vi "multifit_old.vi"(6 "error in":errorcluster, 8 "List Peaks":string[][](table)=[["0", "2.298448", "56622.259938"], ["1", "3.693510", "568942.221745"], ["2", "3.986486", "85674.157303"], ["3", "12.564011", "20786.516854"]], 9 "List Parameter Fit In":dbl[][](array[numeric])=[[61895.26743495138, 2.295902819051137, 0.05132725028401794, 4549.770440475167, 604.272909684641, 0.00013211395312335064, 0.0005412786405150726, 657.5539740905274], [627372.2059878254, 3.692284511840813, 0.05677911685996556, 18601.27709030301, 3836.7824698281233, 8.354403497208279e-05, 0.0003643877607762332, 4160.712473210559], [74116.31578446296, 4.0147483591783155, 0.05085091795005294, 22427.950314927708, 307.3617647197942, 0.00014015981359792937, 0.0002809232075470725, 309.9731656877187], [28273.34836642687, 12.573977083982806, 0.10770256815937904, 51.48314892156685, 1352.5083475039019, 0.0004671472170224425, 0.004032939443201791, 1403.8484860391175]], 10 "List ROI In":dbl[][](array[numeric])=[[2.295902819051137, 0.12087567441886224, 747.0, 785.0, 2.233926550867361, 2.356038682169207, 6063.6329279938445, 123.14309366808929], [3.692284511840813, 0.1337148202052189, 1180.0, 1222.0, 3.625362152280503, 3.760328192140438, 67989.42495261344, 852.13028597231], [4.0147483591783155, 0.11975391177237468, 1283.0, 1320.0, 3.956350297651297, 4.075248951813621, 7193.497223633383, 69.57166423918198], [12.573977083982806, 0.2536395480153376, 3925.0, 4004.0, 12.446356900269128, 12.700221594291389, 5812.069028071378, 495.66499136986374]], 11 "Spectrum In":cluster{"Locations":dbl[], "Amplitudes":dbl[]}={"Locations"=array[8192 elements], "Amplitudes"=array[8192 elements]}) -> (1 "List Parameter Fit Out":dbl[][](array[numeric])=[[72985.42049784464, 2.29530433588858, 0.05722471236395812, -6719.954128683837, 3514.3279732857486, 7.641139969591555e-05, 0.0017646666004499732, 3559.3620345490303], [626906.4516896611, 3.6923878537448513, 0.056725550141628785, 19143.182126509742, 2756.558061175683, 9.742740047455971e-05, 0.00030585131086768315, 3020.7605065816324], [84952.09034117158, 4.0147539339226315, 0.05684400456146576, 11048.984691445543, 3382.5195465814695, 5.6421783276986587e-05, 0.0014333924536871097, 3422.1830799296517]], 2 "List ROI Out":dbl[][](array[numeric])=[[2.29530433588858, 0.13476419761712136, 745.0, 787.0, 2.2274995965883164, 2.3624656364482517, 7971.631104776367, 629.6678820155158], [3.6923878537448513, 0.1335886705835358, 1180.0, 1222.0, 3.625362152280503, 3.760328192140438, 67874.85518278569, 664.4170311995598], [4.0147539339226315, 0.13386763074225186, 1280.0, 1322.0, 3.9467098662327302, 4.0816759060926655, 9216.928010954993, 599.404820008226]], 3 "Spectrum Fitted":cluster{"Array":dbl[], "Array":dbl[]}, 4 "error out":errorcluster)   [LabVIEW 2020]
uses:
  <vilib>/Analysis/6fits.llb/Curve Fitting Criteria.ctl
  <vilib>/gmath/NumericalOptimization/Nonlinear Curve Fit LM bound.vi
  <vilib>/gmath/NI_Gmath.lvlib
  <vilib>/gmath/NumericalOptimization/Nonlinear Curve Fit LM.vi
  <vilib>/Analysis/NI_AALPro.lvlib
panel:
  in  "FWHM Bound Parameters (%)":dbl=60.0
  out "List MultiFit":dbl[][](array[numeric])
  out "R-square":dbl
  out "All FWHM":dbl[](array[numeric])
  out "All Parameters Fit":T1(array[cluster])
  in  "EnOffsetFit":bool
  in  "Erase":bool
  in  "List Fit Peak":T2(array[cluster])
  in  "mapping":u16(ring) items=["Y - Linear", "Y - Log"]
  in  "Fit":bool
  in  "Done":bool
  out "Spectrum":T3(graph)
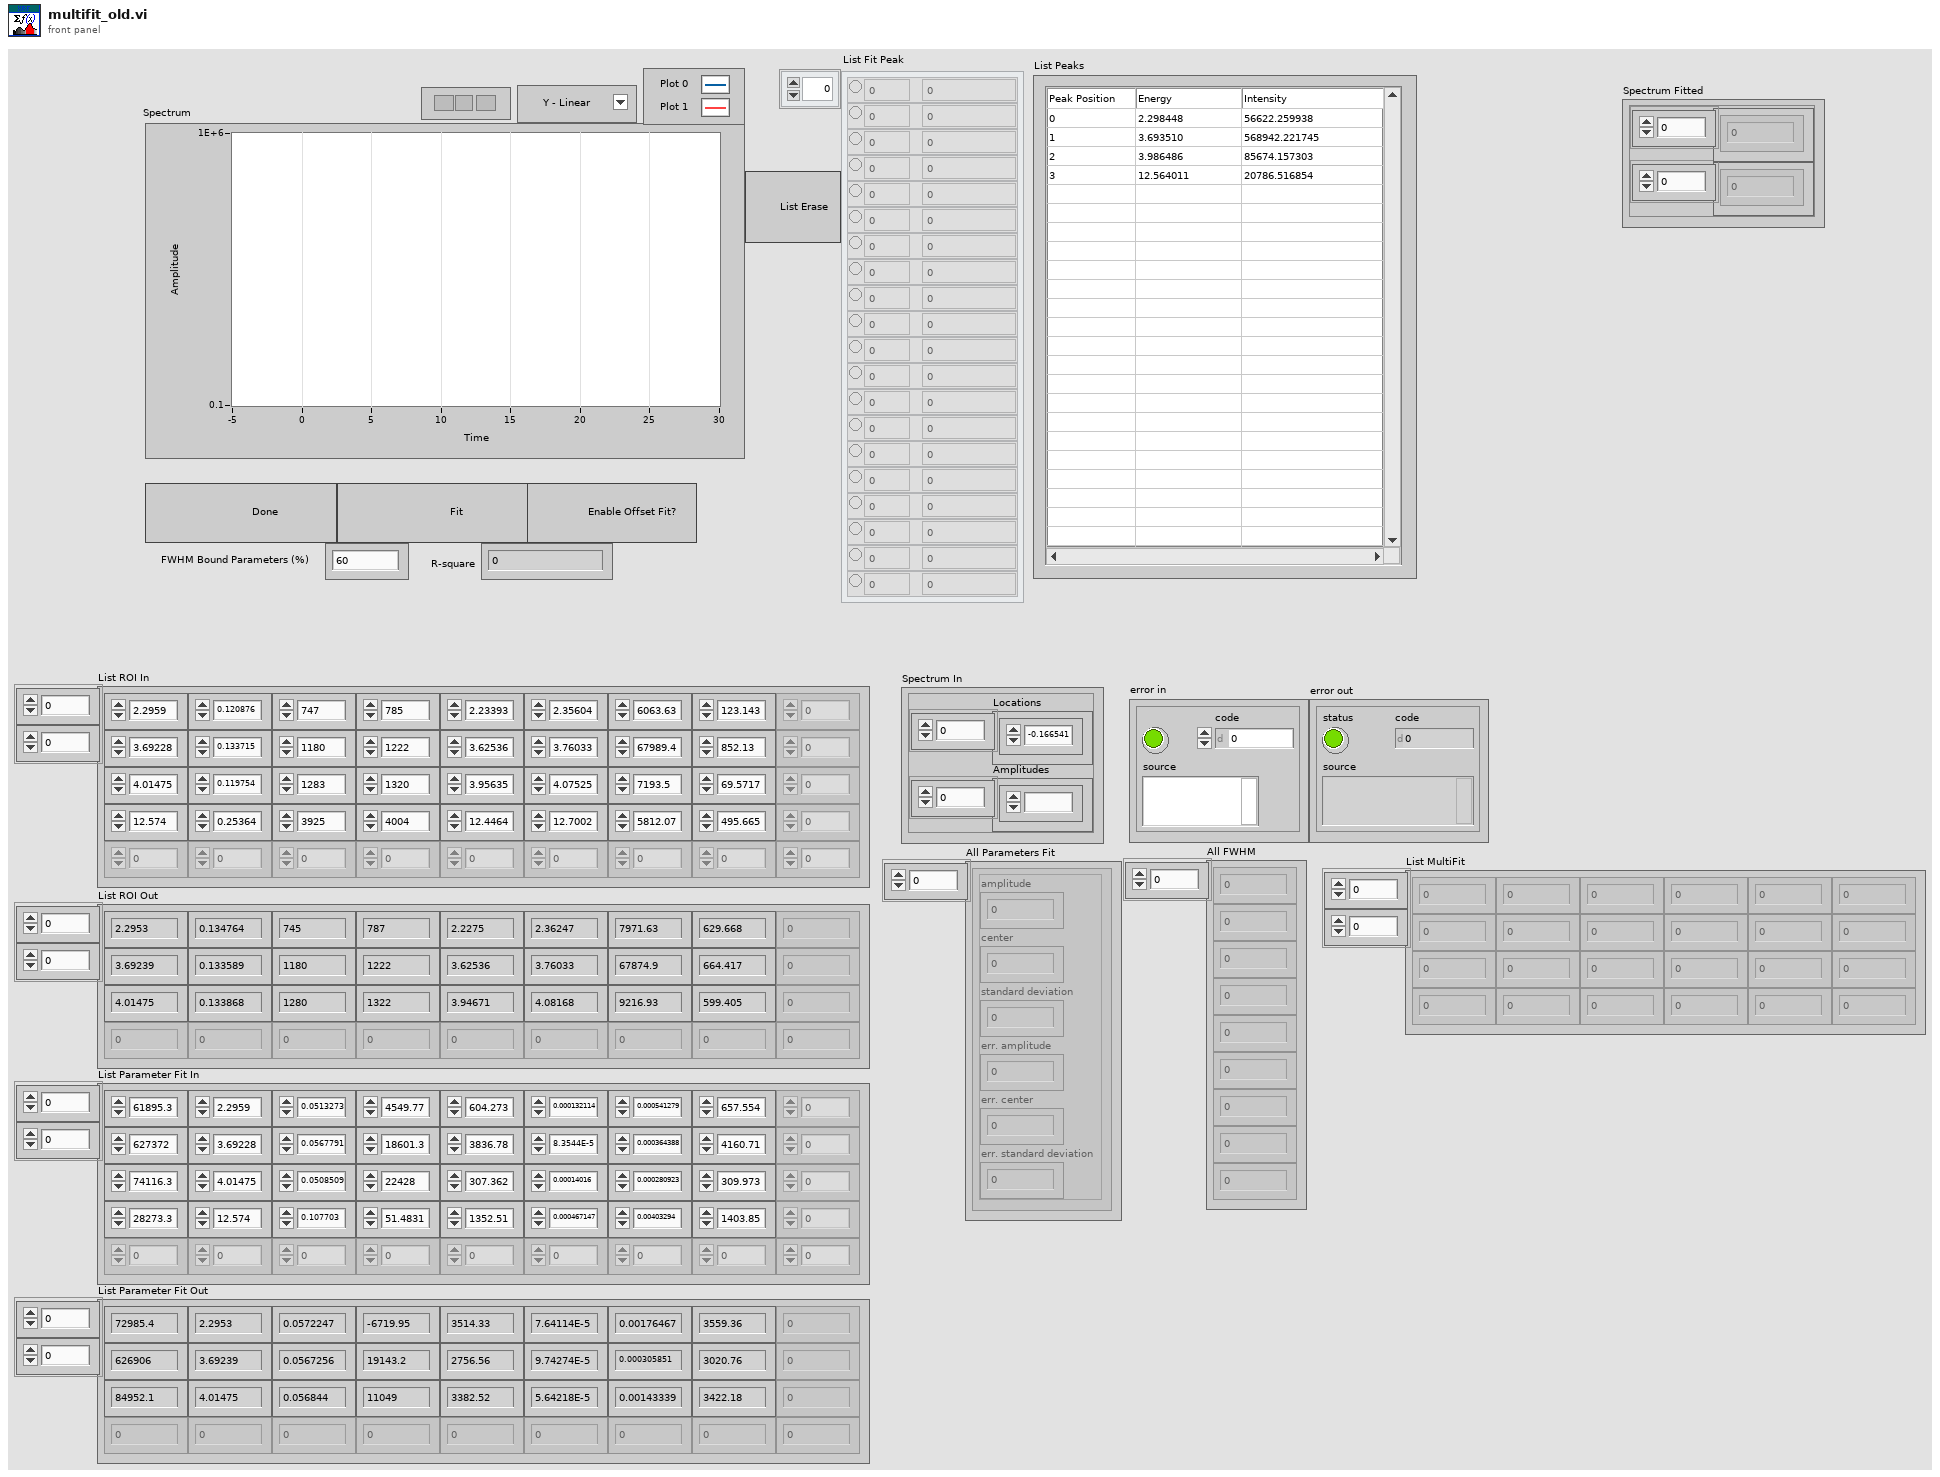
[diagram p1: front panel]
types:
  T1 = cluster{"amplitude":dbl, "center":dbl, "standard deviation":dbl, "err. amplitude":dbl, "err. center":dbl, "err. standard deviation":dbl}[]
  T2 = cluster{"Include":bool, "Position":dbl, "Energy":dbl}[]
  T3 = cluster{"Locations":dbl[], "best nonlinear fit":dbl[]}[]
  T4 = cluster{"Include":bool, "Position":dbl, "Energy":dbl}
  T5 = cluster{"parameter minimum":dbl[], "parameter maximum":dbl[]}
  T6 = typedef "NI_AALPro.lvlib/Curve Fitting Criteria.ctl" = u16
  T7 = typedef "NI_Matrix.lvlib/RealMatrix.ctl" = dbl[][]
  T8 = cluster{"Locations":dbl[], "best nonlinear fit":dbl[]}
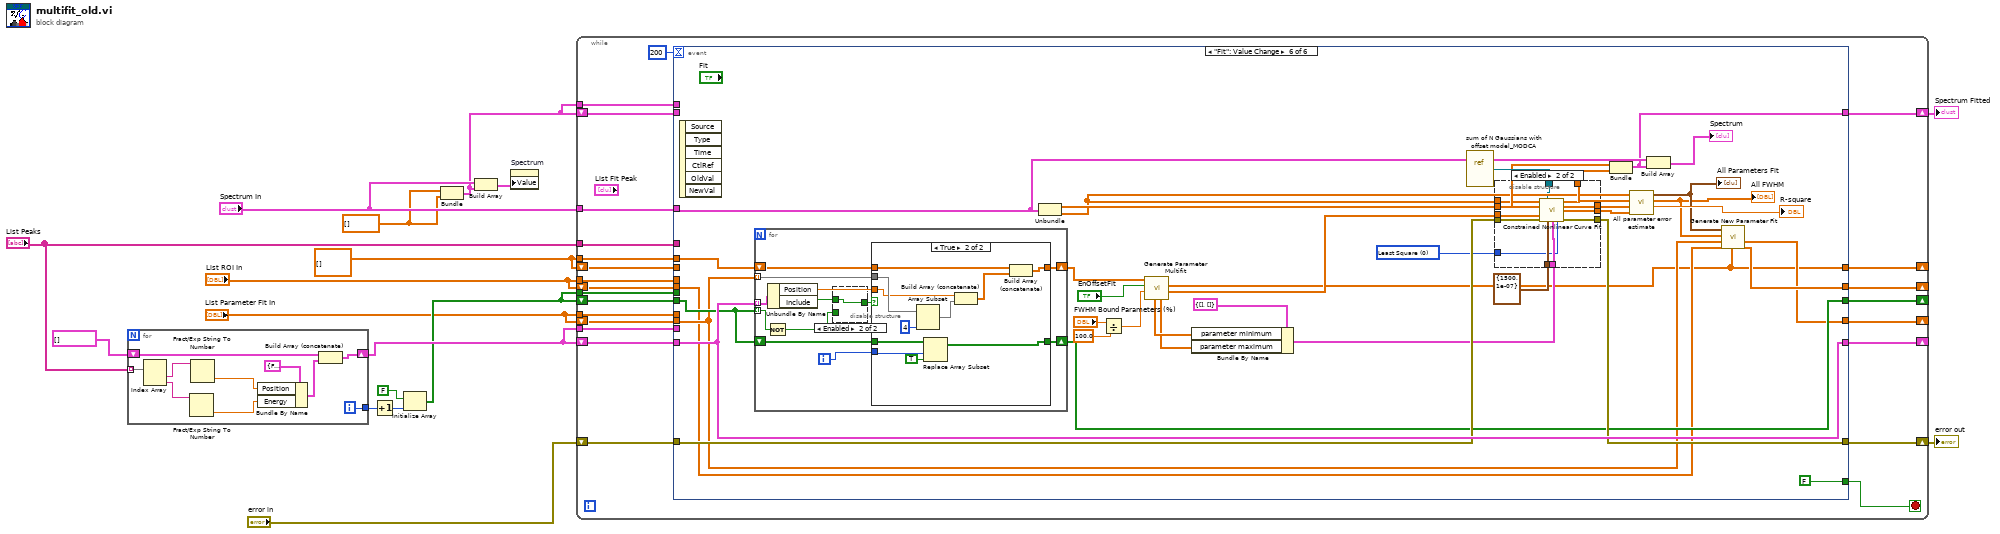
[diagram p0: block diagram]
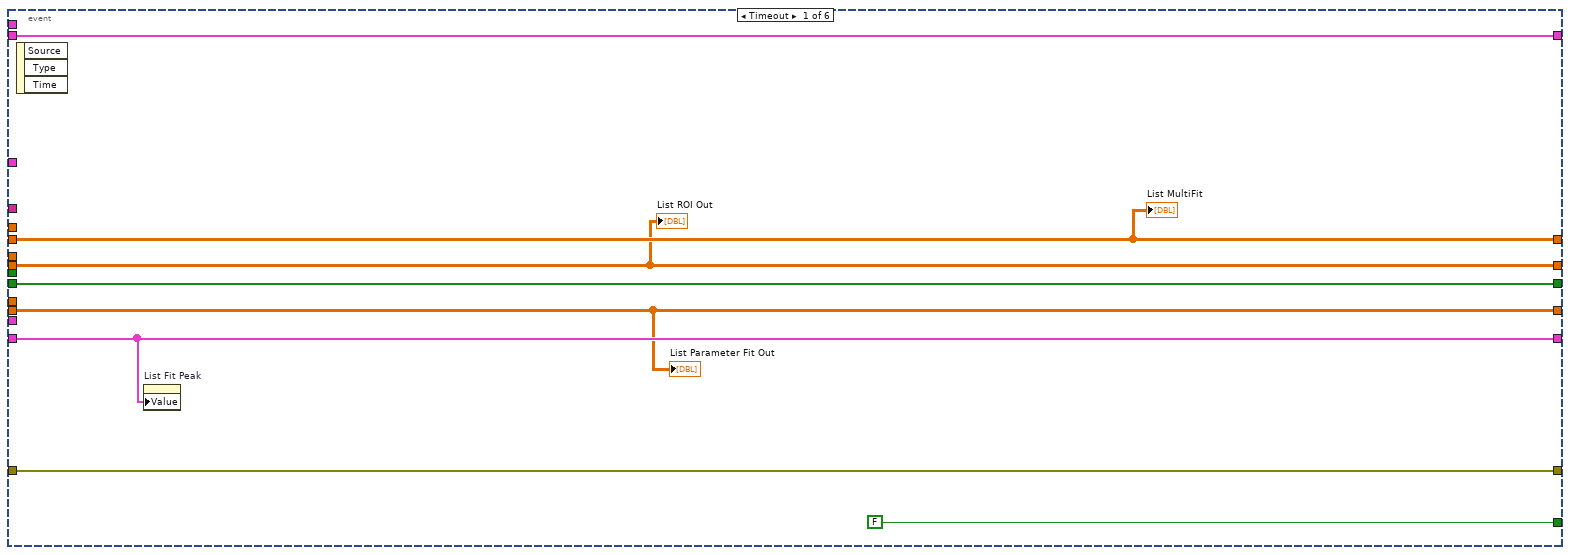
[diagram p2: hidden frame]
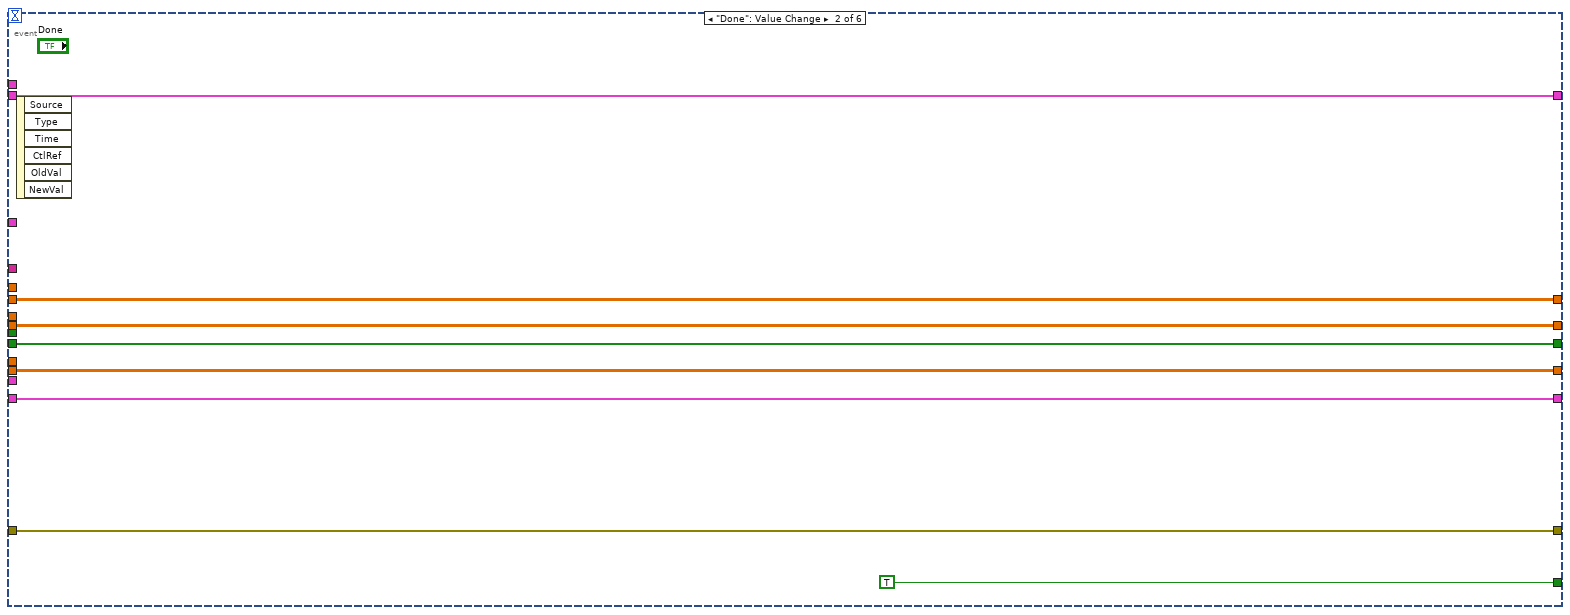
[diagram p3: hidden frame]
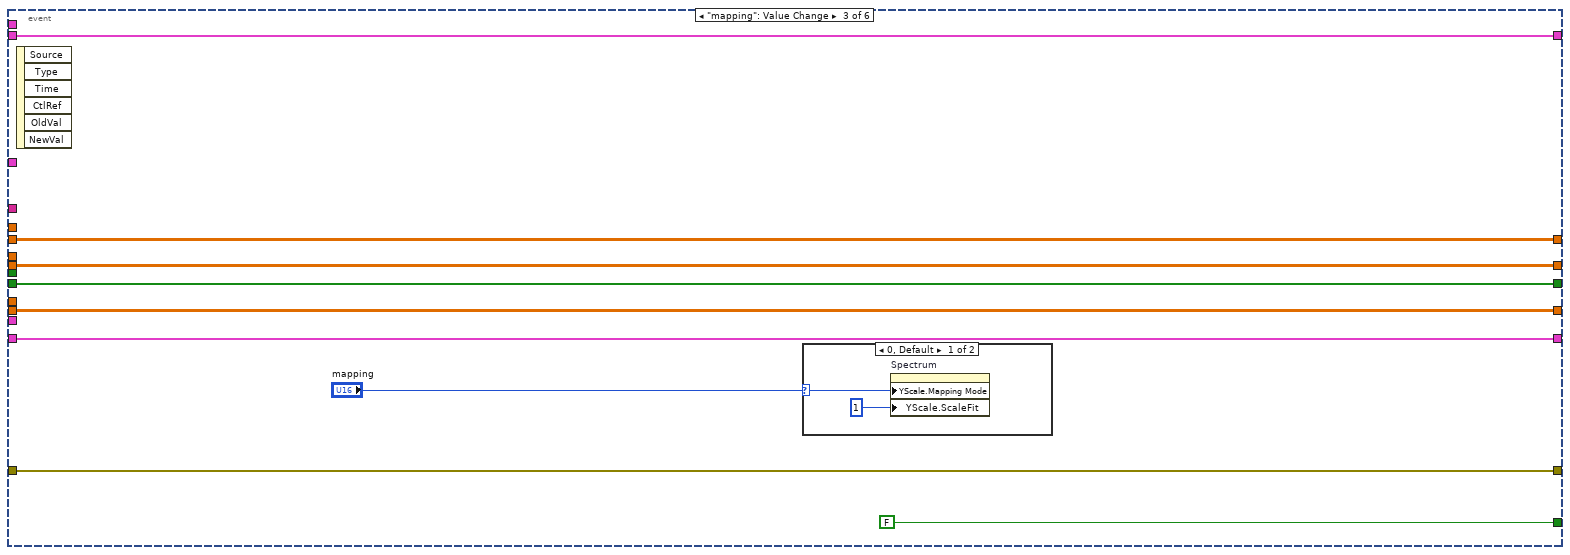
[diagram p4: hidden frame]
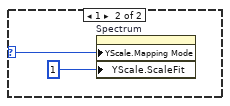
[diagram p5: hidden frame]
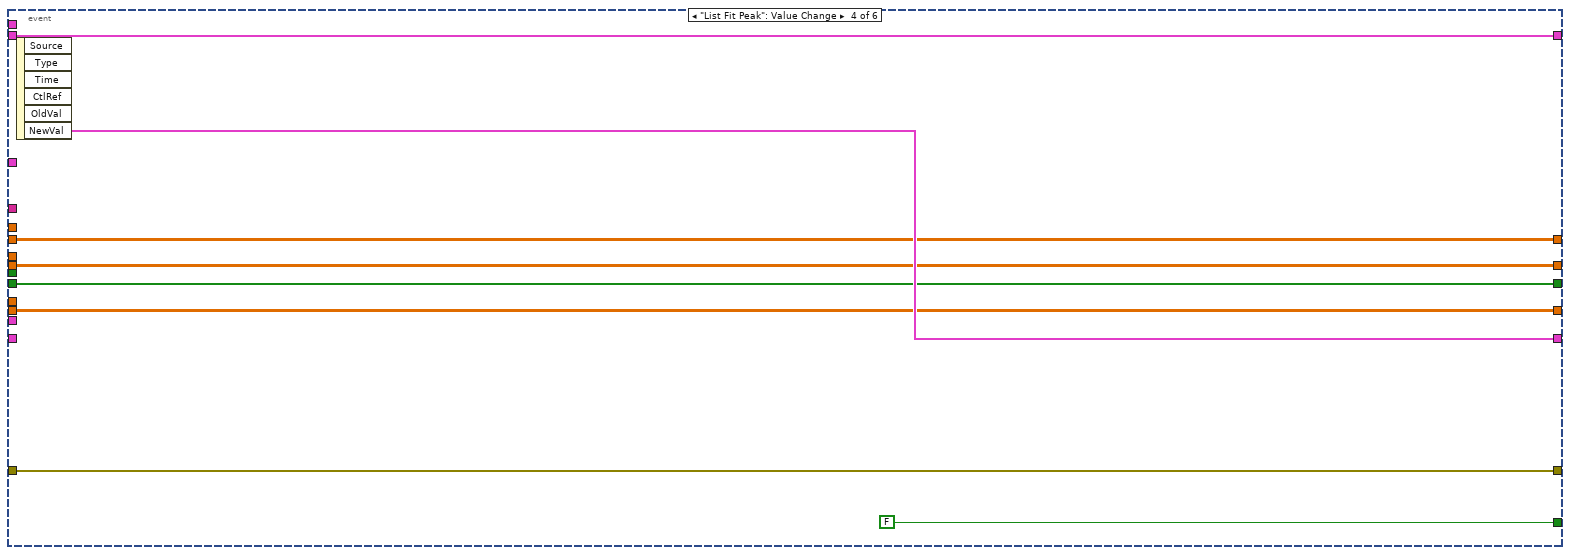
[diagram p6: hidden frame]
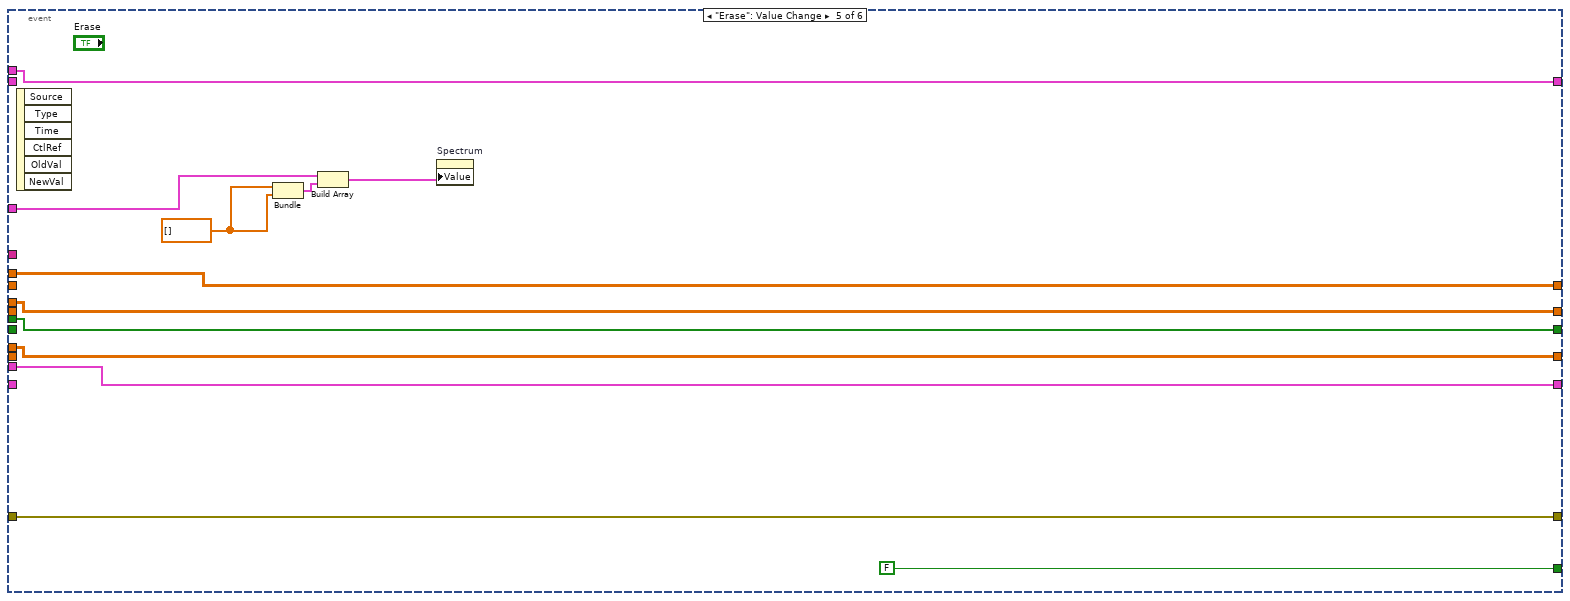
[diagram p7: hidden frame]
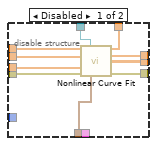
[diagram p8: hidden frame]
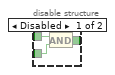
[diagram p9: hidden frame]
diagram:
  w5 = dbl[] []
  w8 = dbl[][] [] ("List ROI In")
  n1 = for {
    tunnel: "List Peaks" -> [w27] mode=indexing
    shift-right: [w23] -> w13
    shift-left: T2 [] ("List Peak") -> [w25]
    tunnel: [w18] -> w12
    i -> [w18]
    n2 = Index Array(array=w27) -> (element #1=w22:string, element #2=w21:string)  [unwired: 2 in]
    n3 = Fract/Exp String To Number(string=w21) -> (number=w19:dbl)  [unwired: 3 in, 1 out]
    n4 = Fract/Exp String To Number(string=w22) -> (number=w20:dbl)  [unwired: 3 in, 1 out]
    n5 = Bundle By Name(cluster=T4 {"Include"=FALSE, "Position"=0.0, "Energy"=0.0} ("Fit Peak Cluster"), "Position"=w20, "Energy"=w19) -> (w24:T4)
    n6 = Build Array (concatenate)(w25, w24) -> (w23:T2)
  }
  n7 = Increment(x=w12) -> (x+1=w11:i32)
  n8 = Initialize Array(FALSE, w11) -> (w9:bool[])
  n9 = Bundle(w5, w5) -> (w2:cluster{dbl[], dbl[]})  [unwired: 1 in]
  n10 = Build Array("Spectrum In", w2) -> (w7:cluster{"Locations":dbl[], "Amplitudes":dbl[]}[])
  n11 = property on="Spectrum" class="XYGraph (strict)"("Value"=w7) -> ()  [unwired: 2 in, 2 out]
  n12 = while {
    shift-right: [w49] -> w16
    shift-left: "error in" -> [w50]
    shift-right: [w47] -> _
    shift-left: w13 -> [w48]
    tunnel: "Spectrum In" -> [w45]
    tunnel: "List Peaks" -> [w44]
    tunnel: "List ROI In" -> [w43]
    tunnel: "List Parameter Fit In" -> [w42]
    tunnel: w13 -> [w41]
    shift-right: [w39] -> _
    shift-left: w8 -> [w40]
    shift-right: [w38] -> _
    shift-left: w9 -> [w37]
    tunnel: w9 -> [w36]
    tunnel: w8 -> [w35]
    shift-right: [w32] -> _
    shift-left: "List ROI In" -> [w34]
    shift-right: [w31] -> _
    shift-left: "List Parameter Fit In" -> [w33]
    shift-right: [w30] -> w1
    shift-left: w2 -> [w29]
    tunnel: w2 -> [w28]
    stop <- w51 stop-if-true
    n13 = event shown="[5] \"Fit\": Value Change" {
      selector: _ -> [_ _ _ _ _ _]
      dyn-events: _ -> [_ _ _ _ _ _]
      timeout: 200 -> [_ _ _ _ _ _]
      tunnel: [FALSE TRUE FALSE FALSE FALSE FALSE] -> w51
      tunnel: w50 -> [w58 w66 w74 w88 w99 w134]
      tunnel: [w58 w66 w74 w88 w99 w133] -> w49
      tunnel: w48 -> [w57 w65 w73 _ _ w135]
      tunnel: [w57 w65 w73 w86 w98 w135] -> w47
      tunnel: w45 -> [_ _ _ _ w92 w128]
      tunnel: w44 -> [_ _ _ _ _ _]
      tunnel: w43 -> [_ _ _ _ w91 _]
      tunnel: w42 -> [_ _ _ _ w90 _]
      tunnel: w41 -> [_ _ _ _ w98 _]
      tunnel: w40 -> [w55 w64 w72 w85 _ _]
      tunnel: [w55 w64 w72 w85 w96 w102] -> w39
      tunnel: [w56 w63 w71 w84 w97 w131] -> w38
      tunnel: w37 -> [w56 w63 w71 w84 _ w132]
      tunnel: w36 -> [_ _ _ _ w97 _]
      tunnel: w35 -> [_ _ _ _ w96 w103]
      tunnel: w34 -> [w54 w62 w69 w83 _ w105]
      tunnel: w33 -> [w53 w61 w70 w82 _ w106]
      tunnel: [w54 w62 w69 w83 w91 w107] -> w32
      tunnel: [w53 w61 w70 w82 w90 w104] -> w31
      tunnel: [w52 w60 w68 w81 w89 w101] -> w30
      tunnel: w29 -> [w52 w60 w68 w81 _ _]
      tunnel: w28 -> [_ _ _ _ w89 _]
      event Timeout {
        n14 = event-data() -> ()  [unwired: 1 in, 3 out]
        n15 = property on="List Fit Peak" class="Arr (strict)"("Value"=w57) -> ()  [unwired: 2 in, 2 out]
        "List MultiFit" <- w55
        "List ROI Out" <- w54
        "List Parameter Fit Out" <- w53
      }
      event "Done": Value Change {
        n16 = event-data() -> ()  [unwired: 1 in, 6 out]
      }
      event "mapping": Value Change {
        n17 = event-data() -> ()  [unwired: 1 in, 6 out]
        n18 = case shown="0, Default" "mapping" {
          selector: "mapping" -> [w78 w80]
          frame 0, Default {
            n19 = property on="Spectrum" class="XYGraph (strict)"("YScale.Mapping Mode"=w78, "YScale.ScaleFit"=u8 1 ("Y Scale.Scale Fit")) -> ()  [unwired: 2 in, 2 out]
          }
          frame 1 {
            n20 = property on="Spectrum" class="XYGraph (strict)"("YScale.Mapping Mode"=w80, "YScale.ScaleFit"=u8 1 ("Y Scale.Scale Fit")) -> ()  [unwired: 2 in, 2 out]
          }
        }
      }
      event "List Fit Peak": Value Change {
        n21 = event-data() -> ("NewVal"=w86:T2)  [unwired: 1 in, 5 out]
      }
      event "Erase": Value Change {
        w95 = dbl[] []
        n22 = event-data() -> ()  [unwired: 1 in, 6 out]
        n23 = Bundle(w95, w95) -> (w93:cluster{dbl[], dbl[]})  [unwired: 1 in]
        n24 = Build Array(w92, w93) -> (w94:cluster{"Locations":dbl[], "Amplitudes":dbl[]}[])
        n25 = property on="Spectrum" class="XYGraph (strict)"("Value"=w94) -> ()  [unwired: 2 in, 2 out]
      }
      event "Fit": Value Change {
        w113 = T6 0 items=["Least Square", "Least Absolute Residual", "Bisquare"] ("method")
        n26 = event-data() -> ()  [unwired: 1 in, 6 out]
        n27 = for {
          tunnel: w106 -> [w167] mode=indexing
          tunnel: w135 -> [w170] mode=indexing
          shift-right: [w169] -> w120
          shift-left: w103 -> [w168]
          tunnel: w132 -> [w166] mode=indexing
          shift-right: [w160] -> w131
          shift-left: w132 -> [w162]
          i -> [w161]
          n28 = Not(x=w166) -> (.not. x?=w163:bool)
          n29 = Unbundle By Name(w170) -> ("Position"=w159:dbl, "Include"=w164:bool)
          n30 = disable-structure shown="Enabled" {
            disable-tunnel: [w173 w174] -> w165
            disable-tunnel: w164 -> [w172 w174]
            disable-tunnel: w163 -> [w171 _]
            frame Disabled {
              n31 = And(x=w172, y=w171) -> (x .and. y?=w173:bool)
            }
            frame Enabled {
            }
          }
          n32 = case shown="True" w165 {
            tunnel: [w176 w187] -> w169
            tunnel: w168 -> [w176 w186]
            tunnel: w167 -> [_ w181]
            tunnel: w162 -> [w175 w185]
            tunnel: w161 -> [_ w180]
            tunnel: [w175 w183] -> w160
            tunnel: w159 -> [_ w178]
            frame False {
            }
            frame True {
              n33 = Array Subset(array=w181, length=4) -> (w179:dbl[])  [unwired: 1 in]
              n34 = Replace Array Subset(array=w185, new element=TRUE ("new element/subarray"), index=w180) -> (w183:bool[])
              n35 = Build Array (concatenate)(w178, w179) -> (w177:dbl[])
              n36 = Build Array (concatenate)(w186, w177) -> (w187:dbl[][])
            }
          }
        }
        n37 = Unbundle(w128) -> ("Locations"=w129:dbl[], "Amplitudes"=w123:dbl[])
        n38 = Divide(x="FWHM Bound Parameters (%)", y=100.0) -> (x/y=w110:dbl)
        n39 = call "Generate Parameter Multifit.vi"("FWHM Bound Parameters (%)"=w110, "EnOffsetFit"="EnOffsetFit", "All Parameter Fit"=w120) -> ("Initial Conditions"=w122:dbl[], "Rearranged Parameter Fit"=w102:dbl[][], "Max Bound Condition"=w115:dbl[], "Min Bound Condition"=w116:dbl[])  [unwired: 4 in, 1 out]
        n40 = Bundle By Name(cluster=T5 {"parameter minimum"=[], "parameter maximum"=[]} ("parameter bounds"), "parameter minimum"=w116, "parameter maximum"=w115) -> (w114:T5)
        n41 = vi-ref "sum of N Gaussians with offset model_MODCA.vi"() -> (w130:refnum<vi>)
        n42 = disable-structure shown="Enabled" {
          disable-tunnel: w134 -> [w146 w157]
          disable-tunnel: [w145 w156] -> w133
          disable-tunnel: w130 -> [w144 w153]
          disable-tunnel: w129 -> [w143 w154]
          disable-tunnel: [w142 w151] -> w126
          disable-tunnel: [w141 w149] -> w125
          disable-tunnel: [w140 w150] -> w124
          disable-tunnel: w123 -> [w139 w155]
          disable-tunnel: w122 -> [w138 w152]
          disable-tunnel: cluster{"max iteration":i32, "tolerance":dbl} {"max iteration"=1500, "tolerance"=1e-07} ("termination") -> [w137 w158]
          disable-tunnel: w114 -> [_ w148]
          disable-tunnel: w113 -> [_ w147]
          frame Disabled {
            n43 = call-poly <vilib>:"Nonlinear Curve Fit.vi"("Y"=w139, "f(x,a)"=w144, "X"=w143, "initial parameters"=w138, "error in (no error)"=w146, "termination"=w137) -> ("best nonlinear fit"=w140:dbl[], "best fit parameters"=w141:dbl[], "covariance"=w142:T7, "error out"=w145:errorcluster)  [unwired: 4 in, 2 out]
          }
          frame Enabled {
            n44 = call-poly <vilib>:"Constrained Nonlinear Curve Fit.vi"("Y"=w155, "f(x,a)"=w153, "X"=w154, "initial parameters"=w152, "error in (no error)"=w157, "termination"=w158, "parameter bounds"=w148, "method"=w147) -> ("best nonlinear fit"=w150:dbl[], "best fit parameters"=w149:dbl[], "covariance"=w151:T7, "error out"=w156:errorcluster)  [unwired: 2 in, 2 out]
          }
        }
        n45 = Bundle("Locations"=w129, "best nonlinear fit"=w124) -> (w101:T8)  [unwired: 1 in]
        n46 = call "All parameter error estimate.vi"("covariance"=w126, "best fit parameters"=w125, "best nonlinear fit"=w124, "Y"=w123) -> ("R-square"=→"R-square":dbl, "All FWHM"=w108:dbl[], "All Parameters Fit"=w109:T1)  [unwired: 4 in, 1 out]
        "All Parameters Fit" <- w109
        "All FWHM" <- w108
        n47 = Build Array(w128, w101) -> (→"Spectrum":T3)
        n48 = call "Generate New Parameter Fit.vi"("Rearranged Parameter Fit"=w102, "List ROI In"=w105, "List MultiFit In"=w106, "All FWHM"=w108, "All Parameters Fit"=w109) -> ("List ROI Out"=w107:dbl[][], "List MultiFit Out"=w104:dbl[][])  [unwired: 5 in]
      }
    }
  }
  "error out" <- w16
  "Spectrum Fitted" <- w1
